vi "XIPIN_Interlaken_1_8.vi"   [LabVIEW 2017]
doc: "The Logicore Interlaken integrated IP core solution is designed to be compliant with Interlaken Protocol Definition, Revision 1.2. Supports different Line rate from 3.125G to 25.78125G with lanes from 1 to 12. Supports AXI4-Lite, IBFC, OOBFC, Duplex, Simplex TX, Simplex RX.\n------------------------------------\n<b>Need License</b> : Yes\n<b>Interface</b> : AXI4"
uses:
  <vilib>/rvi/XilinxIP/XIPIN_XNode/niFpgaXIPIN.xnode
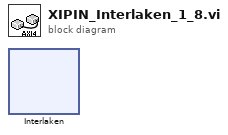
[diagram p0: block diagram]
diagram:
  n1 = xnode ("Interlaken")() -> ()
